vi "TestStepsGui.Results.Update.vi"(7 "Table":refnum<vi>, 8 "error in":errorcluster, 10 "SeqData":T7={"BeginTS"=timestamp(0 s since 1904-01-01), "EndTS"=timestamp(0 s since 1904-01-01), "State"=enum."Init", "Status.Work"=enum."-", "Status.Process"=enum."-", "Status.Home"=enum."-", "Status.Wabco"=enum."-", "Status.Client"=enum."-", "BreakReason"=enum."-", "BreakSource"=enum."-", "DoorLock"=FALSE, "Status.Prod"=[], "UserAction"={"Stop"=FALSE, "Pause"=FALSE, "Next"=FALSE}, "UserData"={"GuiMode"=enum."Process", "Test"={"IgnoreResults"=FALSE, "IgnoreImages"=FALSE, "ServiceMode"=FALSE}, "ContinueOrder"=FALSE}, "Error"={"status"=FALSE, "code"=0, "source"=""}, "Code"={"Ready"=FALSE, "DoubleOrder"=FALSE, "OrderDone"=FALSE, "AllowSingleSlot"=FALSE, "TunedA"=FALSE, "TunedB"=FALSE, "CheckDM"=FALSE, "ThresholdA"=0, "ThresholdB"=0, "Plate"=enum."Wabco", "ImgPath"=path "", "Variant"={"State"=enum."Init", "ImgPath"=path "", "WabcoPlate"="", "WabcoProduct"="", "ClientProduct"="", "ClientPlate"="", "TotalQuantity"=0, "OrderQuantity"=0, "Serial"=0, "Wabco"={"LaserJob"="", "AdditionalTxt"="037", "FactoryCode"="", "RevID"=0, "ForkID"=0, "FailuresLimit"=0, "GlobalCnt"=0, "Bank"=0, "SerialFormat"=enum."6 dig", "CoordA"={"X"=0.0, "Y"=0.0, "Angle"=0.0}, "CoordB"={"X"=0.0, "Y"=0.0, "Angle"=0.0}, "DMCconfig"=0}, "Client"={"LaserJob"="", "AdditionalTxt"="", "FactoryCode"="037", "RevID"=0, "ForkID"=0, "FailuresLimit"=0, "GlobalCnt"=0, "Bank"=0, "SerialFormat"=enum."6 dig", "CoordA"={"X"=0.0, "Y"=0.0, "Angle"=0.0}, "CoordB"={"X"=0.0, "Y"=0.0, "Angle"=0.0}, "DMCconfig"=0}}}, "Rotations"=0, "ProdIdx"=0, "ProdDone"=[], "PrintedSerials-Wabco"=[], "PrintedSerials-Client"=[], "Counters-Wabco"={"Expected"=0, "Done"=0, "OK"=0, "NOK"=0, "NOKlimit"=0, "Part"=0, "PartOK"=0}, "Counters-Client"={"Expected"=0, "Done"=0, "OK"=0, "NOK"=0, "NOKlimit"=0, "Part"=0, "PartOK"=0}}) -> (0 "error out":errorcluster, 1 "changed":bool, 2 "value out":T1)   [LabVIEW 2016]
uses:
  Sequence/Sequence.Data.ctl
  Sequence/Sequence.State.ctl
  Sequence/Sequence.Step.Status.ctl
  Sequence/Sequence.Test.BreakReason.ctl
  Sequence/Sequence.Test.BreakSource.ctl
  Sequence/Sequence.Test.Status.ctl
  Sequence/Sequence.Slot.StatusData.ctl
  Sequence/Sequence.Test.Unload.Status.ctl
  Sequence/Sequence.Prod.StatusData.ctl
  Sequence/Sequence.UserActions.ctl
  Sequence/Sequence.UserData.ctl
  Sequence/Sequence.MainMode.ctl
  MainGui.TestOptions.ctl
  Sequence/Sequence.Code.Sets.ctl
  Sequence/Sequence.PlateType.ctl
  Logger/Logger.Variant.Sets.ctl
  Station/Station.Changeover.State.vi
  Station/Station.Plate.Properties.ctl
  Sequence/Sequence.Code.SerialFormat.ctl
  Drivers/V7310/LowLevel/V7310.Job.Sets.ctl
  Sequence/Sequence.Counters.ctl
  Global/ApplicationGlobal.vi
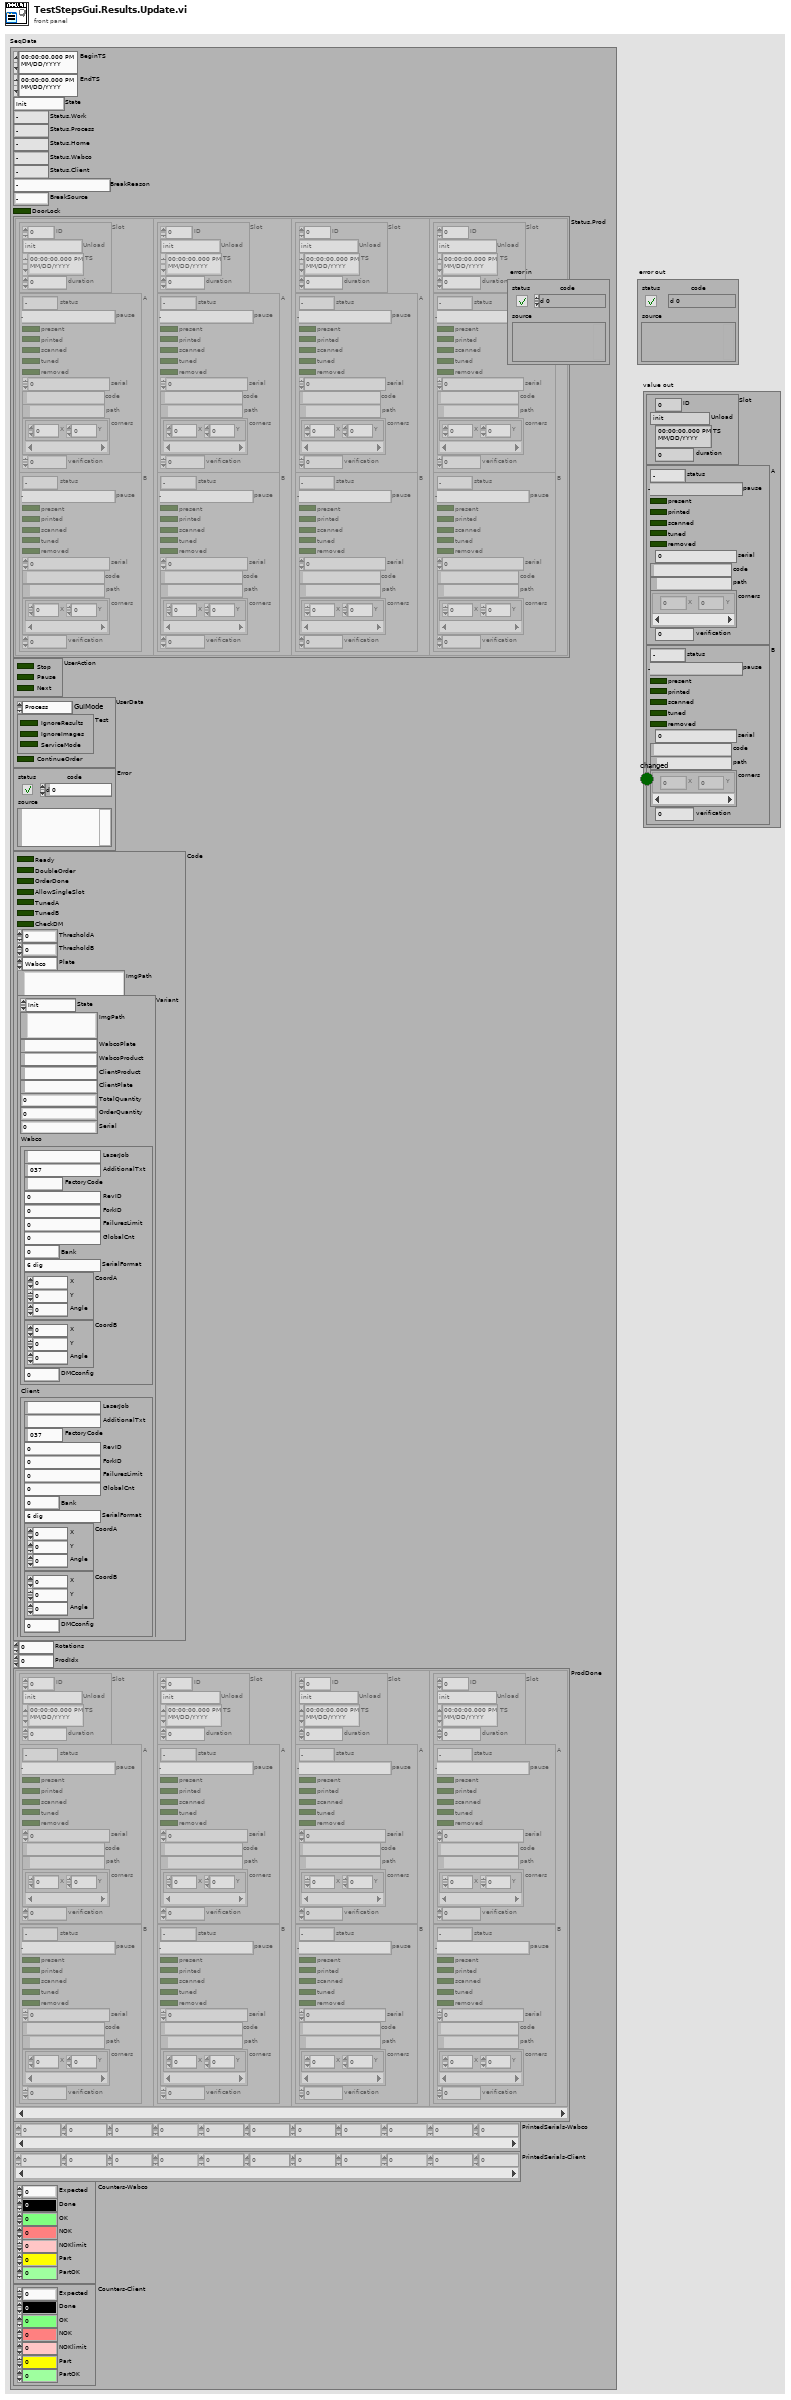
[diagram p1: front panel]
types:
  T1 = typedef "Sequence.Test.Status.ctl" = cluster{"Slot":T2, "A":T4, "B":T4}
  T2 = typedef "Sequence.Slot.StatusData.ctl" = cluster{"ID":i32, "Unload":T3, "TS":timestamp, "duration":u32}
  T3 = typedef "Sequence.Test.Unload.Status.ctl" = enum16{"init", "check NOK", "check OK", "wait on NOK", "wait on OK", "wait on Unload", "done"}
  T4 = typedef "Sequence.Prod.StatusData.ctl" = cluster{"status":T5, "pause":T6, "present":bool, "printed":bool, "scanned":bool, "tuned":bool, "removed":bool, "serial":i32, "code":string, "path":path, "corners":cluster{"X":i32, "Y":i32}[], "verification":u8}
  T5 = typedef "Sequence.Step.Status.ctl" = enum16{"-", "Pending", "Running", "Skipped", "Passed", "Failed", "Done", "Error", "Aborted", "Stopped"}
  T6 = typedef "Sequence.Test.BreakReason.ctl" = enum16{"-", "NOK container", "OK container", "Rev empty", "Rev missing", "Rev wrong", "Fork missing", "Fork wrong", "NOK limit", "Unload failure", "Single slot", "Part done", "Err: Prod move work", "Err: Prod move home", "Err: Prod lift work", "Err: Prod lift home", "Err: Prod Arm Work", "Err: Prod Arm NOK", "Err: Prod Arm OK", "Err: Prod NOK suck", "Err: Prod NOK drop", "Err: Prod OK missing", "Err: Prod OK suck", "Err: Prod OK drop"}
  T7 = typedef "Sequence.Data.ctl" = cluster{"BeginTS":timestamp, "EndTS":timestamp, "State":T8, "Status.Work":T5, "Status.Process":T5, "Status.Home":T5, "Status.Wabco":T5, "Status.Client":T5, "BreakReason":T6, "BreakSource":T9, "DoorLock":bool, "Status.Prod":T1[], "UserAction":T10, "UserData":T11, "Error":errorcluster, "Code":T14, "Rotations":i32, "ProdIdx":i32, "ProdDone":T1[], "PrintedSerials-Wabco":i32[], "PrintedSerials-Client":i32[], "Counters-Wabco":T21, "Counters-Client":T21}
  T8 = typedef "Sequence.State.ctl" = enum16{"Init", "Idle", "Home", "Work", "Run", "Pause"}
  T9 = typedef "Sequence.Test.BreakSource.ctl" = enum16{"-", "A", "B", "A/B"}
  T10 = typedef "Sequence.UserActions.ctl" = cluster{"Stop":bool, "Pause":bool, "Next":bool}
  T11 = typedef "Sequence.UserData.ctl" = cluster{"GuiMode":T12, "Test":T13, "ContinueOrder":bool}
  T12 = typedef "Sequence.MainMode.ctl" = enum16{"Process", "Base", "Order", "Manual", "Logs", "Results", "Stats", "DMC Config"}
  T13 = typedef "MainGui.TestOptions.ctl" = cluster{"IgnoreResults":bool, "IgnoreImages":bool, "ServiceMode":bool}
  T14 = typedef "Sequence.Code.Sets.ctl" = cluster{"Ready":bool, "DoubleOrder":bool, "OrderDone":bool, "AllowSingleSlot":bool, "TunedA":bool, "TunedB":bool, "CheckDM":bool, "ThresholdA":u8, "ThresholdB":u8, "Plate":T15, "ImgPath":path, "Variant":T16}
  T15 = typedef "Sequence.PlateType.ctl" = enum16{"Wabco", "Client"}
  T16 = typedef "Logger.Variant.Sets.ctl" = cluster{"State":T17, "ImgPath":path, "WabcoPlate":string, "WabcoProduct":string, "ClientProduct":string, "ClientPlate":string, "TotalQuantity":u16, "OrderQuantity":u16, "Serial":i32, "Wabco":T18, "Client":T18}
  T17 = typedef "Station.Changeover.State.vi" = enum16{"Init", "Scaning", "NOK", "Wait for ack", "Ready"}
  T18 = typedef "Station.Plate.Properties.ctl" = cluster{"LaserJob":string, "AdditionalTxt":string, "FactoryCode":string, "RevID":u8, "ForkID":u8, "FailuresLimit":u16, "GlobalCnt":i32, "Bank":u8, "SerialFormat":T19, "CoordA":T20, "CoordB":T20, "DMCconfig":i32}
  T19 = typedef "Sequence.Code.SerialFormat.ctl" = enum8{"", "6 dig", "7 dig"}
  T20 = typedef "V7310.Job.Sets.ctl" = cluster{"X":dbl, "Y":dbl, "Angle":dbl}
  T21 = typedef "Sequence.Counters.ctl" = cluster{"Expected":u16, "Done":u16, "OK":u16, "NOK":u16, "NOKlimit":u16, "Part":u16, "PartOK":u16}
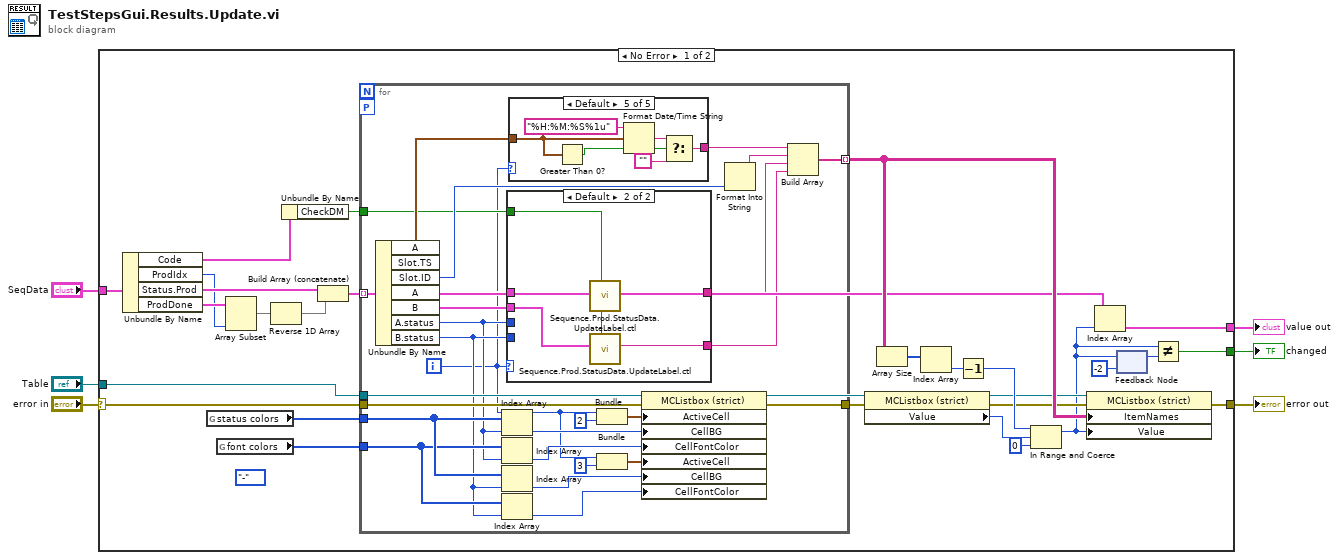
[diagram p0: block diagram]
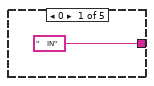
[diagram p2: hidden frame]
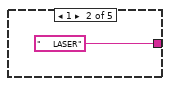
[diagram p3: hidden frame]
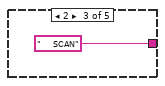
[diagram p4: hidden frame]
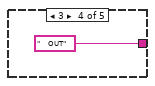
[diagram p5: hidden frame]
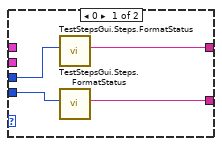
[diagram p6: hidden frame]
diagram:
  n1 = case shown="No Error" "error in" {
    selector: "error in" -> [w22 w80]
    tunnel: "Table" -> [w19 _]
    tunnel: [w20 w80] -> w5
    tunnel: "SeqData" -> [w9 _]
    tunnel: [w11 _] -> w2
    tunnel: [w10 _] -> w1
    frame No Error {
      (unwired) Sequence.Step.Status."-" ("A.status")
      n2 = Unbundle By Name(w9) -> ("Code"=w7:T14, "ProdIdx"=w18:i32, "Status.Prod"=w27:T1[], "ProdDone"=w24:T1[])
      n3 = global read "ApplicationGlobal.vi" "status colors"() -> (w26:u32[])
      n4 = global read "ApplicationGlobal.vi" "font colors"() -> (w25:u32[])
      n5 = Array Subset(array=w24, length=w18) -> (w23:T1[])  [unwired: 1 in]
      n6 = Reverse 1D Array(array=w23) -> (reversed array=w17:T1[])
      n7 = Unbundle By Name(w7) -> ("CheckDM"=w8:bool)
      n8 = Build Array (concatenate)(w27, w17) -> (w13:T1[])
      n9 = for {
        tunnel: w13 -> [w42] mode=indexing
        tunnel: w26 -> [w58]
        tunnel: w25 -> [w57]
        tunnel: [w55] -> w32 mode=indexing
        tunnel: w19 -> [w50]
        tunnel: w22 -> [w49]
        tunnel: [w48] -> w21
        workers-P: _ -> [_]
        tunnel: w8 -> [w38]
        i -> [w34]
        n10 = Unbundle By Name(w42) -> ("Slot.TS"=w40:timestamp, "Slot.ID"=w60:i32, "A"=w59:T4, "B"=w43:T4, "A.status"=w36:T5, "B.status"=w41:T5)  [unwired: 1 out]
        n11 = Index Array(array=w58, index=w36) -> (element=w47:u32)
        n12 = Index Array(array=w57, index=w36) -> (element=w46:u32)
        n13 = Index Array(array=w58, index=w41) -> (element=w45:u32)
        n14 = Index Array(array=w57, index=w41) -> (element=w44:u32)
        n15 = case shown="Default" w34 {
          tunnel: w59 -> [_ w79]
          tunnel: [w74 w78] -> w56
          tunnel: w41 -> [w72 _]
          tunnel: w43 -> [_ w77]
          tunnel: w36 -> [w71 _]
          tunnel: w38 -> [_ w76]
          tunnel: [w73 w75] -> w35
          frame 0 {
            n16 = call "TestStepsGui.Steps.FormatStatus.vi"("Status"=w71) -> ("Status str"=w74:string)  [unwired: 10 in]
            n17 = call "TestStepsGui.Steps.FormatStatus.vi"("Status"=w72) -> ("Status str"=w73:string)  [unwired: 10 in]
          }
          frame Default {
            n18 = call "Sequence.Prod.StatusData.UpdateLabel.ctl"("CheckDM"=w76, "Slot"=w79) -> ("Label"=w78:string)  [unwired: 8 in, 1 out]
            n19 = call "Sequence.Prod.StatusData.UpdateLabel.ctl"("CheckDM"=w76, "Slot"=w77) -> ("Label"=w75:string)  [unwired: 8 in, 1 out]
          }
        }
        n20 = case shown="Default" w34 {
          tunnel: w40 -> [_ _ _ _ w66]
          tunnel: ["    IN" ("date/time string") "    LASER" ("date/time string") "    SCAN" ("date/time string") "    OUT" ("date/time string") w65] -> w39
          frame 0 {
          }
          frame 1 {
          }
          frame 2 {
          }
          frame 3 {
          }
          frame Default {
            n21 = Greater Than 0?(x=w66) -> (x > 0?=w69:bool)
            n22 = Format Date/Time String(time format string (%c)="%H:%M:%S%1u", seconds (now)=w66) -> (date/time string=w68:string)  [unwired: 1 in]
            n23 = Select(t=w68, s=w69, f="") -> (s? t:f=w65:string)
          }
        }
        n24 = Bundle(w34, 2) -> (w51:cluster{i32, i32})  [unwired: 1 in]
        n25 = Bundle(w34, 3) -> (w53:cluster{i32, i32})  [unwired: 1 in]
        n26 = property class="MCListbox (strict)"(reference=w50, error in=w49, "ActiveCell"=w51, "CellBG"=w47, "CellFontColor"=w46, "ActiveCell"=w53, "CellBG"=w45, "CellFontColor"=w44) -> (error out=w48:errorcluster)  [unwired: 1 out]
        n27 = Format Into String(w60) -> (resulting string=w37:string)  [unwired: 3 in, 1 out]
        n28 = Build Array(w39, w37, w56, w35) -> (w55:string[])
      }
      n29 = property class="MCListbox (strict)"(reference=w19, error in=w21) -> (error out=w28:errorcluster, "Value"=w16:i32)  [unwired: 1 out]
      n30 = Array Size(array=w32) -> (size(s)=w31:i32[])
      n31 = Index Array(array=w31) -> (element=w30:i32)  [unwired: 1 in]
      n32 = Decrement(x=w30) -> (x-1=w29:i32)
      n33 = In Range and Coerce(upper limit=w29, x=w16, lower limit=0) -> (coerced(x)=w12:i32)  [unwired: 1 out]
      n34 = property class="MCListbox (strict)"(reference=w19, error in=w28, "ItemNames"=w32, "Value"=w12) -> (error out=w20:errorcluster)  [unwired: 1 out]
      n35 = Index Array(array=w13, index=w12) -> (element=w11:T1)
      n36 = feedback #1(-2 ("ProdNo")) -> (w15:i32)
      n37 = feedback-in #1(w12) -> ()
      n38 = Not Equal?(x=w12, y=w15) -> (x != y?=w10:bool)
    }
    frame Error {
    }
  }
  "error out" <- w5
  "value out" <- w2
  "changed" <- w1
